vi "GetIDNStr.vi"(8 "error in":errorcluster, 11 "Alias":string) -> (0 "error out":errorcluster, 2 "Model ID String":string)   [LabVIEW 2014]
doc: "Displays all hardware and certain properties of that hardware on the specified target."
uses:
  Filter Mode.ctl
  Close (Hardware).vi
  Close (Filter).vi
  Close (System).vi
  nisyscfg.lvlib
  C:/Program Files (x86)/National Instruments/LabVIEW 2014/resource/objmgr/nisysapi.rc
panel:
  out "Intf Type":u16(ring)=1 items=["GPIB"=1, "VXI"=2, "GPIB-VXI"=3, "Serial"=4, "PXI"=5, "TCPIP"=6, "USB"=7, "FireWire"=9]
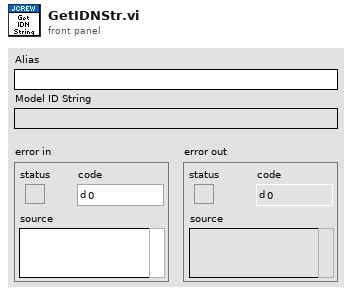
[diagram p1: front panel]
types:
  T1 = typedef "nisyscfg.lvlib/Filter Mode.ctl" = i32
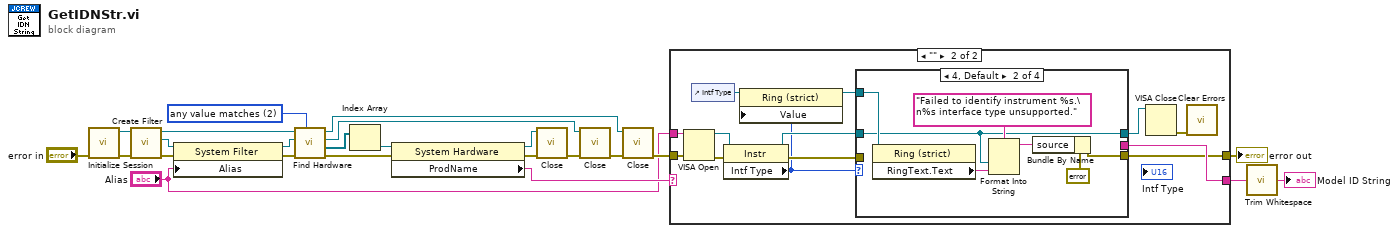
[diagram p0: block diagram]
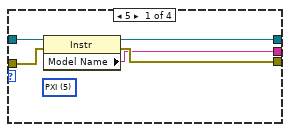
[diagram p3: hidden frame]
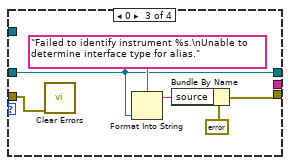
[diagram p4: hidden frame]
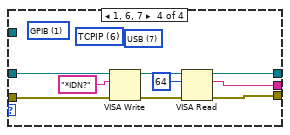
[diagram p5: hidden frame]
diagram:
  w16 = T1 2 items=["all values match"=1, "any value matches"=2, "values do not match"=3, "all properties exist"=4] ("filter mode (all values match)")
  n1 = call "Initialize Session.vi"("error in (no error)"="error in") -> ("error out"=w18:errorcluster, "Session out"=w21:refnum<k21>)  [unwired: 9 in]
  n2 = call "Create Filter.vi"("error in (no error)"=w18, "Session in"=w21) -> ("error out"=w23:errorcluster, "Filter out"=w22:refnum<k20>, "Session out"=w20:refnum<k21>)  [unwired: 7 in]
  n3 = property class="System Filter"(reference=w22, error in=w23, "Alias"="Alias") -> (reference out=w17:refnum<k20>, error out=w19:errorcluster)
  n4 = call "Find Hardware.vi"("Filter Mode (all values match)"=w16, "error in (no error)"=w19, "Filter in"=w17, "Session in"=w20) -> ("error out"=w12:errorcluster, "Resources out"=w10:refnum<k20>[], "Filter out"=w14:refnum<k20>, "Session out"=w24:refnum<k21>)  [unwired: 4 out]
  n5 = Index Array(array=w10) -> (element=w9:refnum<k20>)  [unwired: 1 in]
  n6 = property class="System Hardware"(reference=w9, error in=w12) -> (reference out=w11:refnum<k20>, error out=w7:errorcluster, "ProdName"=w6:string)
  n7 = call-poly "Close.vi"("error in (no error)"=w7, "Resource in"=w11) -> ("error out"=w13:errorcluster)  [unwired: 9 in]
  n8 = call-poly "Close.vi"("error in (no error)"=w13, "Filter in"=w14) -> ("error out"=w15:errorcluster)  [unwired: 9 in]
  n9 = call-poly "Close.vi"("error in (no error)"=w15, "Session in"=w24) -> ("error out"=w5:errorcluster)  [unwired: 9 in]
  n10 = case shown="\"\"" w6 {
    selector: w6 -> [w26 _]
    tunnel: [w26 w30] -> w1
    tunnel: w5 -> [w25 w29]
    tunnel: [w25 w28] -> w4
    tunnel: "Alias" -> [_ w27]
    frame Default {
    }
    frame "" {
      n11 = VISA Open(error in (no error)=w29, VISA resource name=w27) -> (VISA resource name=w39:refnum<visa-resource-name>, error out=w38:errorcluster)  [unwired: 3 in]
      n12 = control-ref of="Intf Type"() -> (w33:refnum<vi>)
      n13 = property class="Instr"(reference=w39, error in=w38) -> (reference out=w37:refnum<visa-resource-name>, error out=w36:errorcluster, "Intf Type"=w32:u16)
      n14 = property class="Ring (strict)"(reference=w33, "Value"=w32) -> (reference out=w31:refnum<vi>)  [unwired: 1 in, 1 out]
      n15 = case shown="4, Default" w32 {
        tunnel: [w43 w45 w53 w66] -> w35
        tunnel: w37 -> [w44 w45 w53 w62]
        tunnel: w36 -> [w40 _ w52 w61]
        tunnel: [w42 w48 w57 w58] -> w28
        tunnel: [w41 _ _ w60] -> w30
        tunnel: w31 -> [_ w46 _ _]
        frame 5 {
          (unwired) u16 5 items=["GPIB"=1, "VXI"=2, "GPIB-VXI"=3, "Serial"=4, "PXI"=5, "TCPIP"=6, "USB"=7, "FireWire"=9] ("Interface Information:Interface Type")
          n16 = property class="Instr"(reference=w44, error in=w40) -> (reference out=w43:refnum<visa-resource-name>, error out=w42:errorcluster, "Model Name"=w41:string)
        }
        frame 4, Default {
          n17 = property class="Ring (strict)"(reference=w46) -> ("RingText.Text"=w47:string)  [unwired: 1 in, 2 out]
          n18 = Format Into String(format string="Failed to identify instrument %s.\n%s interface type unsupported." ("source"), w45, w47) -> (resulting string=w50:string)  [unwired: 2 in, 1 out]
          n19 = Bundle By Name(cluster=errorcluster {"status"=TRUE, "code"=-25, "source"=""} ("error out"), "source"=w50) -> (w48:errorcluster)
        }
        frame 0 {
          n20 = call "Clear Errors.vi"("error in (no error)"=w52) -> ()  [unwired: 5 in, 2 out]
          n21 = Format Into String(format string="Failed to identify instrument %s.\nUnable to determine interface type for alias." ("source"), w53) -> (resulting string=w54:string)  [unwired: 2 in, 1 out]
          n22 = Bundle By Name(cluster=errorcluster {"status"=TRUE, "code"=-25, "source"=""} ("error out"), "source"=w54) -> (w57:errorcluster)
        }
        frame 1, 6, 7 {
          (unwired) u16 6 items=["GPIB"=1, "VXI"=2, "GPIB-VXI"=3, "Serial"=4, "PXI"=5, "TCPIP"=6, "USB"=7, "FireWire"=9] ("Interface Information:Interface Type")
          (unwired) u16 7 items=["GPIB"=1, "VXI"=2, "GPIB-VXI"=3, "Serial"=4, "PXI"=5, "TCPIP"=6, "USB"=7, "FireWire"=9] ("Interface Information:Interface Type")
          (unwired) u16 1 items=["GPIB"=1, "VXI"=2, "GPIB-VXI"=3, "Serial"=4, "PXI"=5, "TCPIP"=6, "USB"=7, "FireWire"=9] ("Interface Information:Interface Type")
          n23 = VISA Write(VISA resource name=w62, write buffer="*IDN?", error in (no error)=w61) -> (VISA resource name out=w64:refnum<visa-resource-name>, error out=w59:errorcluster)  [unwired: 1 out]
          n24 = VISA Read(VISA resource name=w64, byte count=u32 64, error in (no error)=w59) -> (VISA resource name out=w66:refnum<visa-resource-name>, read buffer=w60:string, error out=w58:errorcluster)  [unwired: 1 out]
        }
      }
      n25 = VISA Close(VISA resource name=w35) -> (error out=w34:errorcluster)  [unwired: 1 in]
      n26 = call "Clear Errors.vi"("error in (no error)"=w34) -> ()  [unwired: 5 in, 2 out]
    }
  }
  "error out" <- w4
  n27 = call "Trim Whitespace.vi"("string"=w1) -> ("trimmed string"=→"Model ID String":string)  [unwired: 1 in]
